vi "Image.vi"(2 "XRef":refnum<vi>, 3 "State In":T1={"Input Type"=variant(dbl 0.0), "Width"=0, "Typedef Name"="", "Value Type"=variant, "Selection"=0, "Options"=[], "Selections"=[], "Display Selections"=[], "Element Names"=[], "Typedef Name Width"=0, "Display Selection Width"=[], "Code Generated"=FALSE, "Is DVR"=FALSE, "Write Lock"=FALSE}) -> (0 "Image":picture)   [LabVIEW 2015, in "Read-Write-Signals.xnode"]
doc: "This ability VI is used to describe your XNode's appearance. The origin of Image corresponds to the top-left corner of your XNode. The bounds of your XNode are used to crop this image. If you want LabVIEW to update your image, you need to inform it through the UpdateImage or UpdateImageAndBounds replies. Any areas where you do not draw are transparent, so regions intended to appear white should be explicitly drawn.\n \n Remember to localize any strings that are part of your image.\n\nDefault behavior: None.\n\nThis ability does not provide UI and OS messages are not handled."
uses:
  Read-Write-Signals.xnode
  State.ctl
  Read-Write-Signals Item.ctl
  Read-Write-Signals Sub Item.ctl
  Read-Write-Signals Sub Item Type.ctl
  Read-Write-Signals Selection.ctl
  Read-Write-Signals Display Selection.ctl
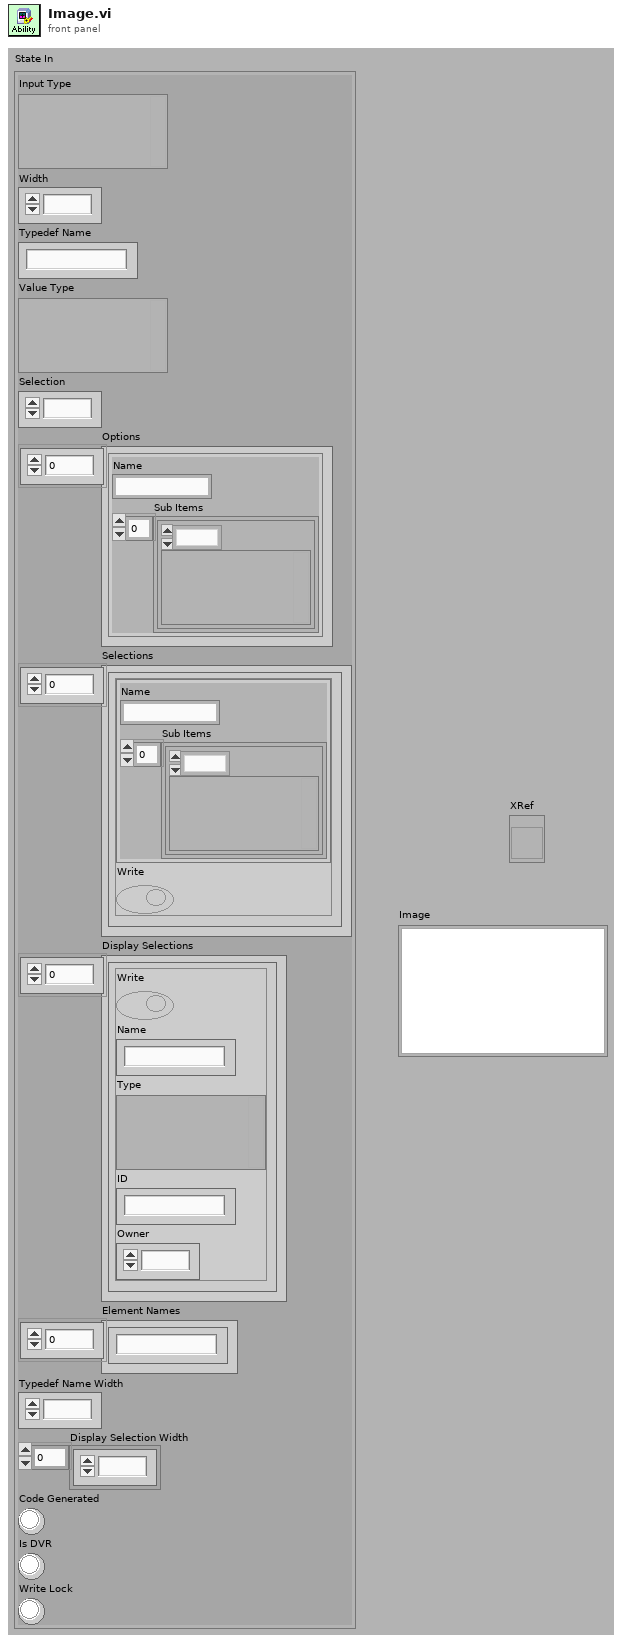
[diagram p1: front panel]
types:
  T1 = typedef "Read-Write-Signals.xnode/State.ctl" = cluster{"Input Type":variant, "Width":i32, "Typedef Name":string, "Value Type":variant, "Selection":i32, "Options":T2[], "Selections":T5[], "Display Selections":T6[], "Element Names":string[], "Typedef Name Width":i32, "Display Selection Width":i32[], "Code Generated":bool, "Is DVR":bool, "Write Lock":bool}
  T2 = typedef "Read-Write-Signals Item.ctl" = cluster{"Name":string, "Sub Items":T3[]}
  T3 = typedef "Read-Write-Signals Sub Item.ctl" = cluster{"Type":T4, "Value":variant}
  T4 = typedef "Read-Write-Signals Sub Item Type.ctl" = enum8{"Cluster Element", "Array Element", "Subarray"}
  T5 = typedef "Read-Write-Signals Selection.ctl" = cluster{"Item":T2, "Write":bool}
  T6 = typedef "Read-Write-Signals Display Selection.ctl" = cluster{"Write":bool, "Name":string, "Type":variant, "ID":string, "Owner":i32}
  T7 = cluster{"horizontal":enum16{"left", "center", "right"}, "vertical":enum16{"top", "center", "bottom"}, "text":enum16{"left", "center", "right"}}
  T8 = enum16{"None", "Stacked", "Clockwise", "Counterclockwise"}
  T9 = cluster{"Font Name:":string, "Size":i16, "Strikeout?":bool, "Italic?":bool, "Underline?":bool, "Outline?":bool, "Shadow?":bool, "Bold?":bool}
  T10 = enum16{"User-specified Font", "Application Font", "System Font", "Dialog Font"}
  T11 = typedef "imagedata.ctl" = cluster{"image type":i32, "image depth":i32, "image":u8[], "mask":u8[], "colors":u32[], "Rectangle":cluster{"left":i16, "top":i16, "right":i16, "bottom":i16}}
  T12 = cluster{"left":i16, "top":i16, "right":i16, "bottom":i16}
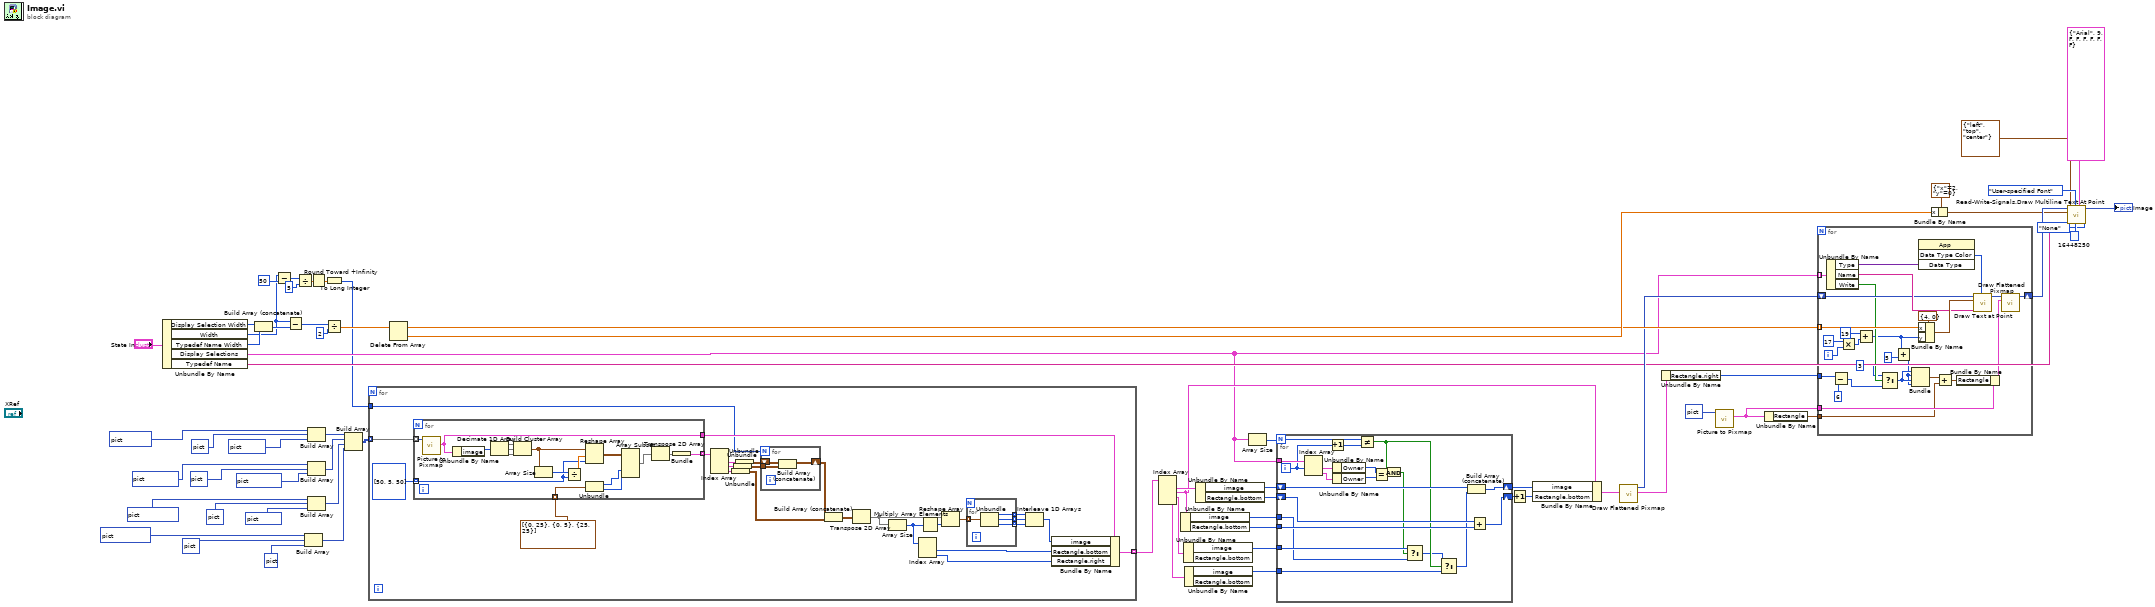
[diagram p0: block diagram]
diagram:
  n1 = Unbundle By Name("State In") -> ("Display Selection Width"=w30:i32[], "Width"=w29:i32, "Typedef Name Width"=w39:i32, "Display Selections"=w24:T6[], "Typedef Name"=w33:string)
  n2 = Build Array (concatenate)(w30, w39) -> (w45:i32[])
  n3 = Subtract(x=w29, y=50) -> (x-y=w50:i32)
  n4 = Subtract(x=w29, y=w45) -> (x-y=w48:i32[])
  n5 = Divide(x=w50, y=i16 5) -> (x/y=w28:dbl)
  n6 = Build Array(picture bytes[2730] ("new picture"), picture bytes[300] ("new picture"), picture bytes[2874] ("new picture")) -> (w16:picture[])
  n7 = Build Array(picture bytes[3032] ("new picture"), picture bytes[315] ("new picture"), picture bytes[3032] ("new picture")) -> (w64:picture[])
  n8 = Build Array(picture bytes[2580] ("new picture"), picture bytes[285] ("new picture"), picture bytes[2580] ("new picture")) -> (w63:picture[])
  n9 = Build Array(picture bytes[2580] ("new picture"), picture bytes[285] ("new picture"), picture bytes[2580] ("new picture")) -> (w62:picture[])
  n10 = Round Toward +Infinity(x=w28) -> (ceil(x): smallest int >= x=w1:dbl)
  n11 = To Long Integer(number=w1) -> (32bit integer=w23:i32)
  n12 = Divide(x=w48, y=i16 2) -> (x/y=w46:dbl[])
  n13 = Build Array(w64, w63, w62, w16) -> (w61:picture[][])
  n14 = for {
    tunnel: w61 -> [w90] mode=indexing
    tunnel: [w71] -> w60 mode=indexing
    tunnel: w23 -> [w67]
    n15 = for {
      tunnel: w90 -> [w114] mode=indexing
      tunnel: i32[] [50, 5, 50] -> [w106] mode=indexing
      tunnel: [w103] -> w88 mode=indexing
      tunnel: [w105] -> w73
      tunnel: cluster{i32, i32}[] [{0, 25}, {0, 5}, {25, 25}] -> [w100] mode=indexing
      n16 = call <vilib>:"Picture to Pixmap.vi"("picture"=w114) -> ("image data"=w105:T11)  [unwired: 9 in, 1 out]
      n17 = Unbundle By Name(w105) -> ("image"=w110:u8[])
      n18 = Decimate 1D Array(w110) -> (w109:u8[], w107:u8[], w108:u8[])
      n19 = Build Cluster Array(w109, w107, w108) -> (w111:cluster{u8, u8, u8}[])
      n20 = Array Size(array=w111) -> (size(s)=w112:i32)
      n21 = Divide(x=w112, y=w106) -> (x/y=w113:dbl)
      n22 = Reshape Array(w111, w113, w106) -> (w102:cluster{u8, u8, u8}[][])
      n23 = Unbundle(w100) -> (w99:i32, w98:i32)
      n24 = Array Subset(array=w102, index (col)=w99, length (col)=w98) -> (w101:cluster{u8, u8, u8}[][])  [unwired: 2 in]
      n25 = Transpose 2D Array(2D array=w101) -> (transposed array=w104:cluster{u8, u8, u8}[][])
      n26 = Bundle(w104) -> (w103:cluster{cluster{u8, u8, u8}[][]})  [unwired: 1 in]
    }
    n27 = Index Array(array=w88) -> (element #1=w86:cluster{cluster{u8, u8, u8}[][]}, element #2=w87:cluster{cluster{u8, u8, u8}[][]}, element #3=w84:cluster{cluster{u8, u8, u8}[][]})  [unwired: 3 in]
    n28 = Unbundle(w84) -> (w68:cluster{u8, u8, u8}[][])
    n29 = Unbundle(w87) -> (w69:cluster{u8, u8, u8}[][])
    n30 = Unbundle(w86) -> (w70:cluster{u8, u8, u8}[][])
    n31 = for {
      N: w67 -> [_]
      shift-right: [w95] -> w85
      shift-left: w70 -> [w96]
      tunnel: w69 -> [w97]
      n32 = Build Array (concatenate)(w96, w97) -> (w95:cluster{u8, u8, u8}[][])
    }
    n33 = Build Array (concatenate)(w85, w68) -> (w83:cluster{u8, u8, u8}[][])
    n34 = Transpose 2D Array(2D array=w83) -> (transposed array=w74:cluster{u8, u8, u8}[][])
    n35 = Array Size(array=w74) -> (size(s)=w82:i32[])
    n36 = Index Array(array=w82) -> (element #1=w75:i32, element #2=w72:i32)  [unwired: 2 in]
    n37 = Multiply Array Elements(1:w82) -> (0:w81:i32)
    n38 = Reshape Array(w74, w81) -> (w80:cluster{u8, u8, u8}[])
    n39 = for {
      tunnel: w80 -> [w94] mode=indexing
      tunnel: [w93] -> w79 mode=indexing
      tunnel: [w92] -> w78 mode=indexing
      tunnel: [w91] -> w77 mode=indexing
      n40 = Unbundle(w94) -> (w93:u8, w92:u8, w91:u8)
    }
    n41 = Interleave 1D Arrays(w79, w78, w77) -> (w76:u8[])
    n42 = Bundle By Name(cluster=w73, "image"=w76, "Rectangle.bottom"=w75, "Rectangle.right"=w72) -> (w71:T11)
  }
  n43 = Delete From Array(array=w46) -> (deleted portion=w38:dbl, array with subset deleted=w37:dbl[])  [unwired: 2 in]
  n44 = Index Array(array=w60) -> (element #1=w59:T11, element #2=w54:T11, element #3=w27:T11, element #4=w15:T11)  [unwired: 4 in]
  n45 = Unbundle By Name(w54) -> ("image"=w57:u8[], "Rectangle.bottom"=w56:i16)
  n46 = Unbundle By Name(w27) -> ("image"=w26:u8[])  [unwired: 1 out]
  n47 = Unbundle By Name(w15) -> ("image"=w14:u8[])  [unwired: 1 out]
  n48 = Unbundle By Name(w59) -> ("image"=w58:u8[], "Rectangle.bottom"=w55:i16)
  n49 = Array Size(array=w24) -> (size(s)=w25:i32)
  n50 = for {
    N: w25 -> [w121]
    tunnel: w57 -> [w123]
    tunnel: w56 -> [w134]
    shift-right: [w131] -> w52
    shift-left: w58 -> [w135]
    shift-right: [w132] -> w53
    shift-left: w55 -> [w133]
    tunnel: w24 -> [w130]
    tunnel: w26 -> [w124]
    tunnel: w14 -> [w117]
    i -> [w119]
    n51 = Index Array(array=w130, index #1=w119) -> (element #1=w129:T6, element #2=w128:T6)  [unwired: 1 in]
    n52 = Increment(x=w119) -> (x+1=w120:i32)
    n53 = Unbundle By Name(w129) -> ("Owner"=w127:i32)
    n54 = Unbundle By Name(w128) -> ("Owner"=w126:i32)
    n55 = Not Equal?(x=w121, y=w120) -> (x != y?=w118:bool)
    n56 = Equal?(x=w127, y=w126) -> (x = y?=w125:bool)
    n57 = And(x=w118, y=w125) -> (x .and. y?=w122:bool)
    n58 = Select(t=w124, s=w122, f=w123) -> (s? t:f=w116:u8[])
    n59 = Select(t=w116, s=w118, f=w117) -> (s? t:f=w115:u8[])
    n60 = Build Array (concatenate)(w135, w115) -> (w131:u8[])
    n61 = Add(x=w133, y=w134) -> (x+y=w132:i16)
  }
  n62 = Increment(x=w53) -> (x+1=w13:i16)
  n63 = Bundle By Name(cluster=w54, "image"=w52, "Rectangle.bottom"=w13) -> (w34:T11)
  n64 = call <vilib>:"Draw Flattened Pixmap.vi"("image data"=w34) -> ("new picture"=w36:picture)  [unwired: 1 in, 7 out]
  n65 = Unbundle By Name(w34) -> ("Rectangle.right"=w41:i16)
  n66 = call <vilib>:"Picture to Pixmap.vi"("picture"=picture bytes[84] ("new picture")) -> ("image data"=w31:T11)  [unwired: 9 in, 1 out]
  n67 = Unbundle By Name(w31) -> ("Rectangle"=w40:T12)
  n68 = for {
    tunnel: w24 -> [w157] mode=indexing
    shift-right: [w152] -> w44
    shift-left: w36 -> [w155]
    tunnel: w37 -> [w154] mode=indexing
    tunnel: w41 -> [w150]
    tunnel: w40 -> [w144]
    tunnel: w31 -> [w151]
    i -> [w161]
    n69 = Unbundle By Name(w157) -> ("Type"=w136:variant, "Name"=w156:string, "Write"=w148:bool)
    n70 = Subtract(x=w150, y=i16 6) -> (x-y=w147:i16)
    n71 = Multiply(x=17, y=w161) -> (x*y=w159:i32)
    n72 = Add(x=19, y=w159) -> (x+y=w140:i32)
    n73 = Select(t=i16 3 ("y"), s=w148, f=w147) -> (s? t:f=w145:i16)
    n74 = Add(x=w140, y=5) -> (x+y=w139:i32)
    n75 = Bundle("y"=w145, w139, "y"=w145, w139) -> (w143:cluster{"y":i16, i32, "y":i16, i32})  [unwired: 1 in]
    n76 = invoke class="App" method="Data Type Color"("Data Type"=w136) -> ("Data Type Color"=w137:u32)  [unwired: 3 in, 3 out]
    n77 = Bundle By Name(cluster=cluster{"x":i16, "y":i16} {"x"=4, "y"=0} ("origin"), "x"=w154, "y"=w140) -> (w162:cluster{"x":i16, "y":i16})
    n78 = Add(x=w143, y=w144) -> (x+y=w142:cluster{i16, i32, i16, i32})
    n79 = Bundle By Name(cluster=w151, "Rectangle"=w142) -> (w141:T11)
    n80 = call <vilib>:"Draw Text at Point.vi"("text color(black)"=w137, "text"=w156, "origin"=w162, "picture"=w155) -> ("new picture"=w153:picture)  [unwired: 6 in, 1 out]
    n81 = call <vilib>:"Draw Flattened Pixmap.vi"("image data"=w141, "picture"=w153) -> ("new picture"=w152:picture)  [unwired: 7 out]
  }
  n82 = Bundle By Name(cluster=cluster{"x":i16, "y":i16} {"x"=2, "y"=0} ("origin"), "x"=w38) -> (w42:cluster{"x":i16, "y":i16})
  n83 = call "Read-Write-Signals.Draw Multiline Text At Point.vi"("text orientation"=T8."None", "[user-specified font]"=T9 {"Font Name:"="Arial", "Size"=9, "Strikeout?"=FALSE, "Italic?"=FALSE, "Underline?"=FALSE, "Outline?"=FALSE, "Shadow?"=FALSE, "Bold?"=FALSE}, "text color(black)"=u32 16448250, "desired font(Application)"=T10."User-specified Font", "text"=w33, "alignment(left, top,text)"=T7 {"horizontal"=enum."left", "vertical"=enum."top", "text"=enum."center"}, "origin"=w42, "picture"=w44) -> ("new picture"=→"Image":picture)  [unwired: 2 in, 1 out]
